vi "散斑图像作用及差分.vi"(5 "散斑矩阵":dbl[][](array[numeric]), 6 "散斑行数":i32, 7 "图像连接一维数组":dbl[](array[numeric])) -> (0 "照射差分求和数组":dbl[](array[numeric]), 1 "散斑行求和一维数组":dbl[](array[numeric]), 2 "照射差分求和均值":dbl, 3 "照射结果求和数组":dbl[](array[numeric]), 4 "照射结果均值":dbl)   [LabVIEW 2018]
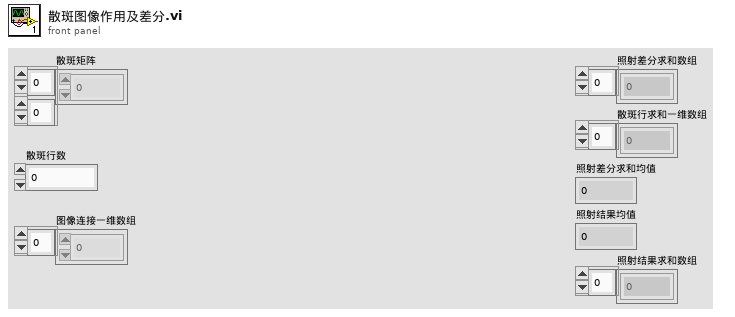
[diagram p1: front panel]
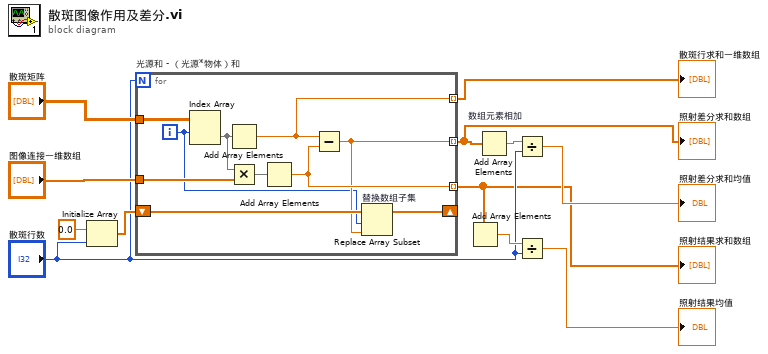
[diagram p0: block diagram]
diagram:
  n1 = Initialize Array(0.0 ("元素"), "散斑行数") -> (w8:dbl[])
  n2 = for "光源和 - （光源*物体）和" {
    N: "散斑行数" -> [_]
    tunnel: "散斑矩阵" -> [w22]
    tunnel: "图像连接一维数组" -> [w21]
    shift-right: [w17] -> _
    shift-left: w8 -> [w18]
    tunnel: [w15] -> w1 mode=indexing
    tunnel: [w16] -> w3 mode=indexing
    tunnel: [w13] -> w2 mode=indexing
    i -> [w14]
    n3 = Index Array(array=w22, index (row)=w14) -> (element=w19:dbl[])  [unwired: 1 in]
    n4 = Add Array Elements(numeric array=w19) -> (sum=w13:dbl)
    n5 = Multiply(x=w19, y=w21) -> (x*y=w20:dbl[])
    n6 = Add Array Elements(numeric array=w20) -> (sum=w16:dbl)
    n7 = Subtract(x=w13, y=w16) -> (x-y=w15:dbl)
    n8 = Replace Array Subset "替换数组子集"(array=w18, new element=w15, index=w14) -> (w17:dbl[])
  }
  "照射差分求和数组" <- w1
  "散斑行求和一维数组" <- w2
  "照射结果求和数组" <- w3
  n9 = Add Array Elements(numeric array=w3) -> (sum=w6:dbl)
  n10 = Add Array Elements "数组元素相加"(numeric array=w1) -> (sum=w11:dbl)
  n11 = Divide(x=w11, y="散斑行数") -> (x/y=→"照射差分求和均值":dbl)
  n12 = Divide(x=w6, y="散斑行数") -> (x/y=→"照射结果均值":dbl)
